vi "Get Audio Device Info.vi"(8 "error in (no error)":errorcluster, 9 "Device Type (Playback)":T2=enum."Playback", 10 "Playback Device ID":u8[](array[numeric]), 11 "Backend (Default)":T5) -> (0 "error out":errorcluster, 3 "Device Info":T1)   [LabVIEW 2020, in "G-Audio.lvlib"]
doc: "Get basic audio information about the file."
uses:
  G-Audio.lvlib
  Controls/Backends.ctl
  Controls/Audio Device Type.ctl
  Controls/Audio Device Info.ctl
  Controls/Audio Device Format.ctl
  <vilib>/Utility/file.llb/Application Directory.vi
  <vilib>/Utility/error.llb/Error Cluster From Error Code.vi
  Controls/Audio Device Native Data Format.ctl
  lib/g_audio_32.dll
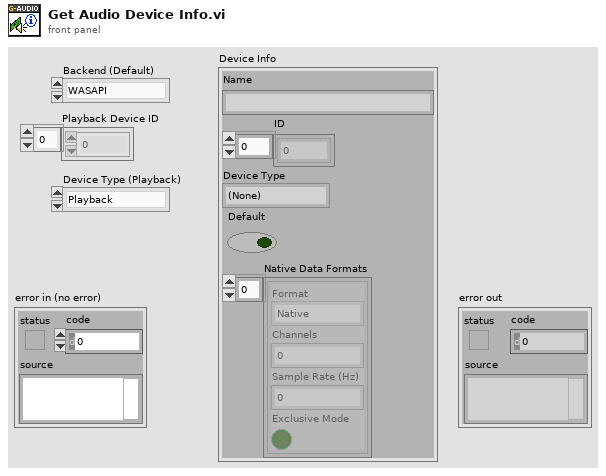
[diagram p1: front panel]
types:
  T1 = typedef "G-Audio.lvlib/Audio Device Info.ctl" = cluster{"Name":string, "ID":u8[], "Device Type":T2, "Default":bool, "Native Data Formats":T3[]}
  T2 = typedef "G-Audio.lvlib/Audio Device Type.ctl" = enum16{"(None)", "Playback", "Capture", "Duplex", "Loopback"}
  T3 = typedef "G-Audio.lvlib/Audio Device Native Data Format.ctl" = cluster{"Format":T4, "Channels":u32, "Sample Rate (Hz)":u32, "Exclusive Mode":bool}
  T4 = typedef "G-Audio.lvlib/Audio Device Format.ctl" = enum16{"Native", "U8", "I16", "I32", "SGL"}
  T5 = typedef "G-Audio.lvlib/Backends.ctl" = enum16{"WASAPI", "DirectSound", "WinMM", "Core Audio", "sndio", "audio(4)", "OSS", "PulseAudio", "ALSA", "JACK", "AAudio", "OpenSL|ES", "Web Audio", "Custom", "Null", "Default"}
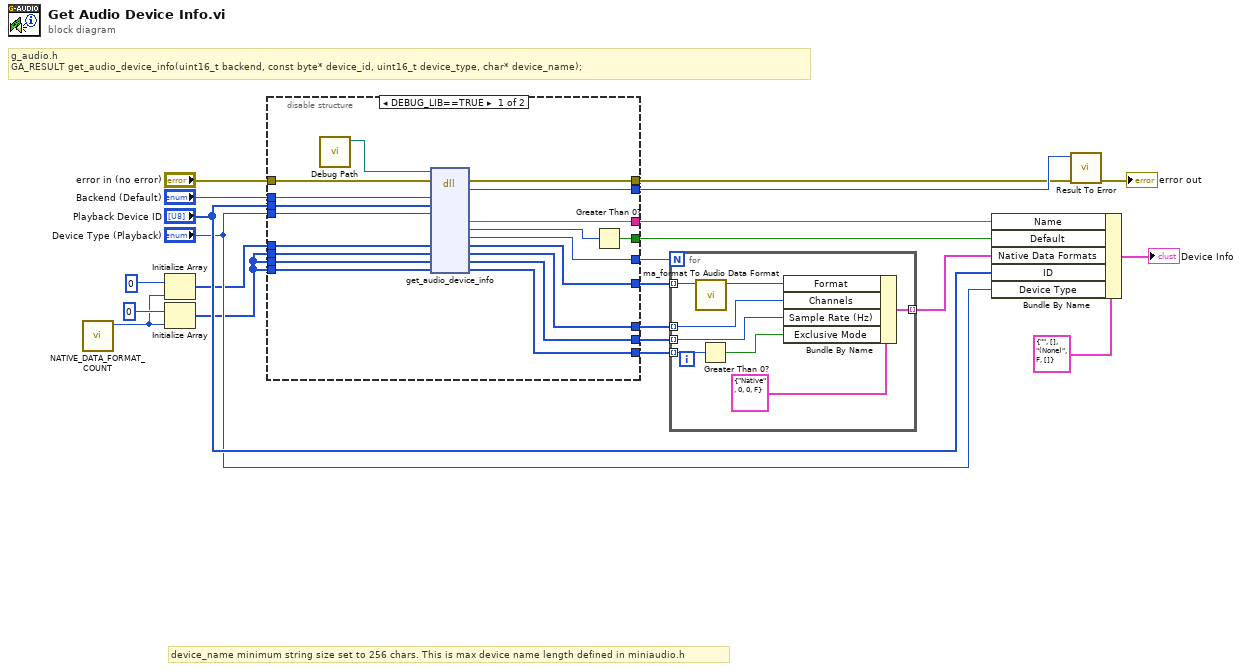
[diagram p0: block diagram]
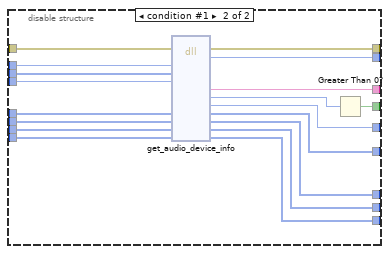
[diagram p2: hidden frame]
diagram:
  # "device_name minimum string size set to 256 chars. This is max device name length defined in miniaudio.h"
  # "g_audio.h\nGA_RESULT get_audio_device_info(uint16_t backend, const byte* device_id, uint16_t device_type, char* device_name);"
  n1 = call "NATIVE_DATA_FORMAT_COUNT.vi"() -> ("NATIVE_DATA_FORMAT_COUNT"=w3:i32)  [unwired: 11 in]
  n2 = Initialize Array(u16 0 ("element"), w3) -> (w2:u16[])
  n3 = Initialize Array(u32 0 ("element"), w3) -> (w1:u32[])
  n4 = disable-structure shown="DEBUG_LIB==TRUE" {
    disable-tunnel: "error in (no error)" -> [w40 w59]
    disable-tunnel: [w24 w57] -> w21
    disable-tunnel: [w23 w58] -> w20
    disable-tunnel: "Backend (Default)" -> [w39 w56]
    disable-tunnel: "Playback Device ID" -> [w38 w55]
    disable-tunnel: "Device Type (Playback)" -> [w37 w54]
    disable-tunnel: [w32 w53] -> w13
    disable-tunnel: [w30 w51] -> w12
    disable-tunnel: [w29 w50] -> w11
    disable-tunnel: [w28 w49] -> w10
    disable-tunnel: [w27 w48] -> w8
    disable-tunnel: [w26 w47] -> w7
    disable-tunnel: [w25 w46] -> w6
    disable-tunnel: w2 -> [w36 w45]
    disable-tunnel: w1 -> [w35 w44]
    disable-tunnel: w1 -> [w34 w43]
    disable-tunnel: w1 -> [w33 w42]
    frame condition #0 (active) {
      n5 = call "Debug Path.vi"() -> ("Debug Path"=w41:path)  [unwired: 11 in]
      n6 = dll-call lib="?" fn="get_audio_device_info"(path in=w41, error in=w40, "backend_in"=w39, "device_id"=w38, "device_type"=w37, "device_native_data_format"=w36, "device_native_data_channels"=w35, "device_native_data_sample_rate"=w34, "device_native_data_exclusive_mode"=w33) -> (error out=w23:errorcluster, "result"=w24:i32, "device_name"=w32:string, "device_default"=w31:u32, "device_native_data_format_count"=w29:u32, "device_native_data_format"=w28:u16[], "device_native_data_channels"=w27:u32[], "device_native_data_sample_rate"=w26:u32[], "device_native_data_exclusive_mode"=w25:u32[])  [unwired: 7 in, 1 out]
      n7 = Greater Than 0?(x=w31) -> (x > 0?=w30:bool)
    }
    frame condition #1 {
      n8 = dll-call lib="C:/github/dataflowg/g-audio/src/LabVIEW/G-Audio/lib/g_audio_*.*" fn="get_audio_device_info"(error in=w59, "backend_in"=w56, "device_id"=w55, "device_type"=w54, "device_native_data_format"=w45, "device_native_data_channels"=w44, "device_native_data_sample_rate"=w43, "device_native_data_exclusive_mode"=w42) -> (error out=w58:errorcluster, "result"=w57:i32, "device_name"=w53:string, "device_default"=w52:u32, "device_native_data_format_count"=w50:u32, "device_native_data_format"=w49:u16[], "device_native_data_channels"=w48:u32[], "device_native_data_sample_rate"=w47:u32[], "device_native_data_exclusive_mode"=w46:u32[])  [unwired: 8 in, 1 out]
      n9 = Greater Than 0?(x=w52) -> (x > 0?=w51:bool)
    }
  }
  n10 = for {
    N: w11 -> [_]
    tunnel: w10 -> [w67] mode=indexing
    tunnel: [w64] -> w9 mode=indexing
    tunnel: w8 -> [w63] mode=indexing
    tunnel: w7 -> [w62] mode=indexing
    tunnel: w6 -> [w61] mode=indexing
    n11 = call "ma_format To Audio Data Format.vi"("ma_format"=w67) -> ("Format"=w65:T4)  [unwired: 10 in]
    n12 = Greater Than 0?(x=w61) -> (x > 0?=w60:bool)
    n13 = Bundle By Name(cluster=T3 {"Format"=enum."Native", "Channels"=0, "Sample Rate (Hz)"=0, "Exclusive Mode"=FALSE} ("Native Data Format"), "Format"=w65, "Channels"=w63, "Sample Rate (Hz)"=w62, "Exclusive Mode"=w60) -> (w64:T3)
  }
  n14 = Bundle By Name(cluster=T1 {"Name"="", "ID"=[], "Device Type"=enum."(None)", "Default"=FALSE, "Native Data Formats"=[]} ("Audio Device Info"), "Name"=w13, "Default"=w12, "Native Data Formats"=w9, "ID"="Playback Device ID", "Device Type"="Device Type (Playback)") -> (→"Device Info":T1)
  n15 = call "Result To Error.vi"("error in (no error)"=w20, "Result Code"=w21) -> ("error out"=→"error out":errorcluster)  [unwired: 9 in]
